vi "Fetch Waveforms.vi"(8 "error in":errorcluster, 11 "Fetch Display CFG in":refnum<class "Fetch Display CFG.lvclass">) -> (0 "error out":errorcluster, 2 "Last Waveforms":map{u8, waveform(dbl)}(c390), 3 "Fetch Display out":refnum<class "Fetch Display CFG.lvclass">)   [LabVIEW 2023, in "OWON SDS1022.lvlib" / "Fetch Display CFG.lvclass"]
doc: "Since more than one Channel could be configured for Acquisition one has to specify\nwhich specific channel data to fetch"
uses:
  Fetch Display CFG.lvclass
  HAL/Scope VISA/Configuration/Scope VISA CFG.lvclass/Scope VISA CFG.ctl
  8256a423-1469-4ca0-9fd9-6d00fd4a7322.vi
  df7a16ed-28d0-4fb1-a819-19d595bd8faa.vi
  2b215bc2-ab3d-4632-bf26-83ca2c28cad1.vi
  <vilib>/JDP Science/JSONtext/Find Item.vi
  <vilib>/JDP Science/JSONtext/Next JSON Value.vi
  <vilib>/JDP Science/JSONtext/String Subset.vi
  <vilib>/JDP Science/JSONtext/Parsing/Advance past next JSON Value (inlined COPY).vi
  <vilib>/JDP Science/JSONtext/Parsing/Advance past whitespace.vi
  <vilib>/JDP Science/JSONtext/Parsing/Advance past String.vi
  <vilib>/JDP Science/JSONtext/Parsing/Advance past Number.vi
  <vilib>/JDP Science/JSONtext/Parsing/Advance past Line Ending.vi
  <vilib>/JDP Science/JSONtext/Parsing/Parse Full Path or Item Name.vi
  <vilib>/JDP Science/JSONtext/Parsing/Advance past Array.vi
  <vilib>/JDP Science/JSONtext/Parsing/Advance past Object.vi
  <vilib>/JDP Science/JSONtext/support/Error Cluster From Code.vi
  <vilib>/JDP Science/JSONtext/Offset/Find Item Locations by Path.vi
  <vilib>/JDP Science/JSONtext/JSON text to Variant.vi
  <vilib>/JDP Science/JSONtext/LVClass Serializer/JSONtext LVClass Serializer.lvclass
  Fetch Display CFG.lvclass/Fetch Display CFG.ctl
  HAL/Scope VISA/Configuration/Scope VISA CFG.lvclass
  OWON SDS1022.lvlib
  D:/git/OWON-SDS1022-LabVIEW/OWON SDS1022/Configurations/SDS1000 Base CFG/SDS1022 Base CFG.lvclass
  D:/git/HAL/Scope VISA/Configuration/Scope VISA CFG.lvclass
  D:/git/HAL/Configuration Base/Configuration Base.lvclass
  D:/git/HAL/Interfaces/IConfigure/IConfigure.lvclass
  D:/git/HAL/Interfaces/IConfigure Scope/IConfigure Scope.lvclass
  D:/git/OWON-SDS1022-LabVIEW/OWON SDS1022/Configurations/Fetch Display CFG/Fetch Display CFG.lvclass
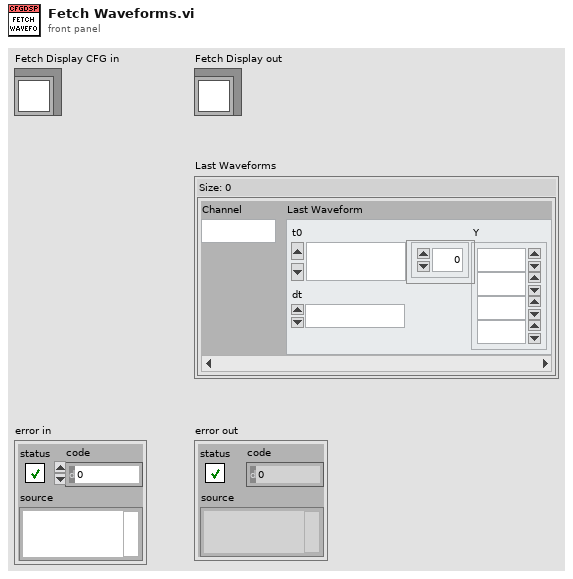
[diagram p1: front panel]
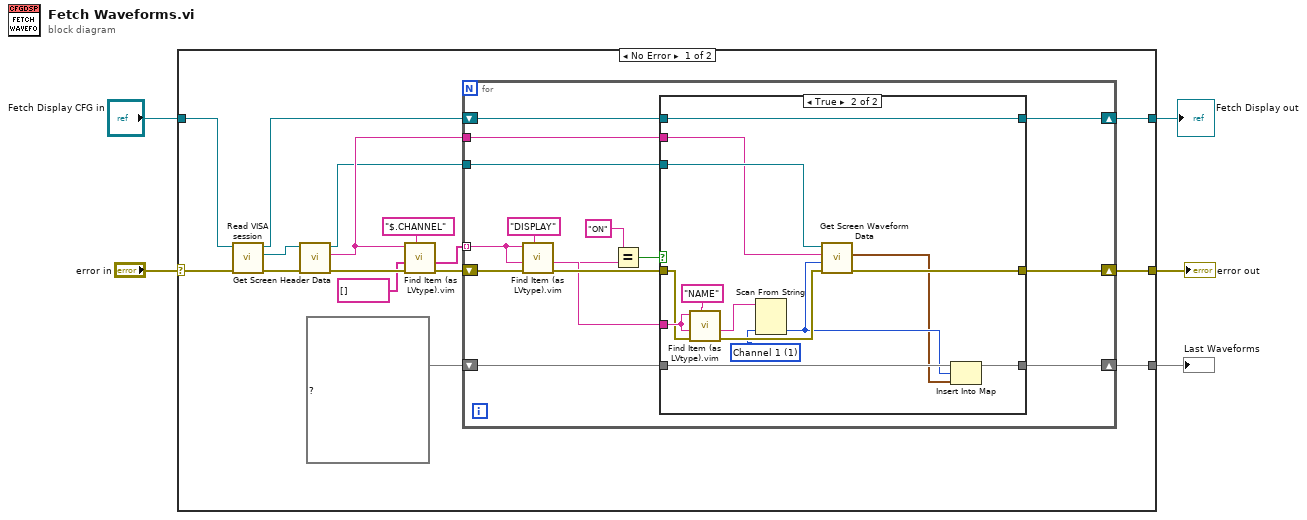
[diagram p0: block diagram]
diagram:
  n1 = case shown="No Error" "error in" {
    selector: "error in" -> [w20 w54]
    tunnel: "Fetch Display CFG in" -> [w21 w53]
    tunnel: [w16 w53] -> w4
    tunnel: [w15 w54] -> w3
    tunnel: [w14 _] -> w1
    frame No Error {
      n2 = call "Read VISA session.vi"("error in (no error)"=w20, "Scope VISA CFG in"=w21) -> ("error out"=w19:errorcluster, "VISA session"=w8:refnum<visa-resource-name>, "Scope VISA CFG out"=w7:refnum<class "Fetch Display CFG.lvclass">)  [unwired: 7 in]
      n3 = call "Get Screen Header Data.vi"("error in"=w19, "VISA session"=w8) -> ("error out"=w18:errorcluster, "Head JSON"=w9:string, "VISA session out"=w6:refnum<visa-resource-name>)  [unwired: 7 in]
      n4 = call "Find Item (as LVtype).vim"("$Path or Item Name"="$.CHANNEL", "error in (no error)"=w18, "Data Type and Default Value"=string[] [], "JSON"=w9) -> ("error out"=w12:errorcluster, "Data"=w10:string[])  [unwired: 4 in, 2 out]
      n5 = for {
        tunnel: w6 -> [w35]
        shift-right: [w30] -> w15
        shift-left: w12 -> [w27]
        tunnel: w10 -> [w26] mode=indexing
        shift-right: [w32] -> w16
        shift-left: w7 -> [w33]
        shift-right: [w28] -> w14
        shift-left: map{u8, waveform(dbl)} {} ("map") -> [w29]
        tunnel: w9 -> [w22]
        n6 = call "Find Item (as LVtype).vim"("$Path or Item Name"="DISPLAY" ("element"), "error in (no error)"=w27, "Data Type and Default Value"=w26, "JSON"=w26) -> ("error out"=w31:errorcluster, "Data"=w24:string)  [unwired: 4 in, 2 out]
        n7 = Equal?(x="ON", y=w24) -> (x = y?=w23:bool)
        n8 = case shown="True" w23 {
          tunnel: w35 -> [_ w45]
          tunnel: w33 -> [w37 w42]
          tunnel: [w37 w42] -> w32
          tunnel: w31 -> [w38 w47]
          tunnel: [w38 w52] -> w30
          tunnel: w29 -> [w36 w51]
          tunnel: [w36 w50] -> w28
          tunnel: w26 -> [_ w48]
          tunnel: w22 -> [_ w39]
          frame False {
          }
          frame True {
            w44 = u8 1 items=["Channel 1"=1, "Channel 2"=2] ("Channel")
            n9 = call "Find Item (as LVtype).vim"("$Path or Item Name"="NAME", "error in (no error)"=w47, "Data Type and Default Value"=w48, "JSON"=w48) -> ("error out"=w46:errorcluster, "Data"=w43:string)  [unwired: 4 in, 2 out]
            n10 = Scan From String(input string=w43, default 1=w44) -> (output 1=w41:u8)  [unwired: 3 in, 3 out]
            n11 = call "Get Screen Waveform Data.vi"("error in"=w46, "Channel"=w41, "Screen Head"=w39, "VISA Refnum in"=w45) -> ("error out"=w52:errorcluster, "Waveform"=w40:waveform(dbl))  [unwired: 5 in, 1 out]
            n12 = Insert Into Map(map in=w51, key=w41, value=w40) -> (map out=w50:map{u8, waveform(dbl)})  [unwired: 2 out]
          }
        }
      }
    }
    frame Error {
    }
  }
  "error out" <- w3
  "Fetch Display out" <- w4
  "Last Waveforms" <- w1
